vi "QueryFirst.vi"(6 "commandTimeout in":i32=-1, 7 "CommandType":i32(ring)=-1 items=["Text"=1, "StoredProcedure"=4, "TableDirect"=512], 8 "error in (no error)":errorcluster, 9 "DynamicParameters in":refnum<class "DynamicParameters.lvclass">, 10 "sql":string, 11 "ADOMapper in":refnum<class "ADOMapper.lvclass">) -> (0 "error out":errorcluster, 2 "Value":variant, 3 "ADOMapper out":refnum<class "ADOMapper.lvclass">)   [LabVIEW 2020, in "ORM_ADONet.lvlib" / "ADOMapper.lvclass"]
uses:
  ADOMapper.lvclass
  C:/Program Files/National Instruments/LabVIEW 2020/vi.lib/Viviota/shared/ORM.lvlibp/ORM/SqlMapper/SqlMapper.lvclass
  <vilib>/Viviota/shared/ORM.lvlibp/ORM/DynamicParameters/DynamicParameters.lvclass
  <vilib>/Viviota/shared/ORM_DBC_dotNet.lvlibp/dbcDotNet/ORM_DBC_dotNet.lvclass
  System.Data
  <vilib>/Viviota/shared/ORM.lvlibp/ORM/SqlMapper/Read DbConnection.vi
  <vilib>/Viviota/shared/ORM_DBC_dotNet.lvlibp/dbcDotNet/Read transaction.vi
  <vilib>/Viviota/shared/ORM.lvlibp/ORM/DbConnection/DbConnection.lvclass
  ADORow/ADORow.lvclass
  <userlib>/_OpenG.lib/error/error.llb/openg_error.lvlib
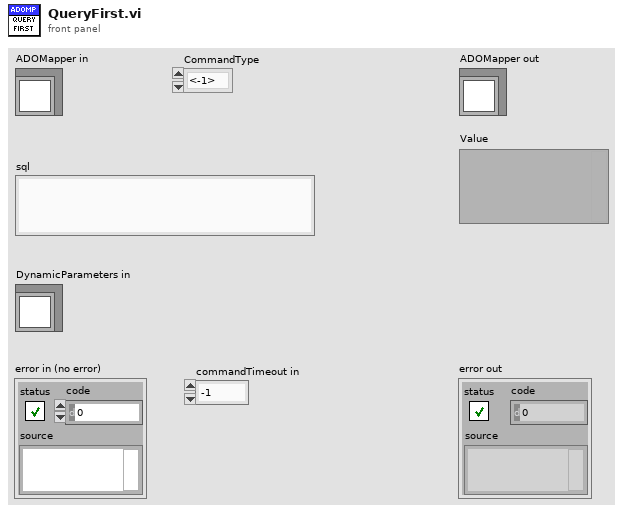
[diagram p1: front panel]
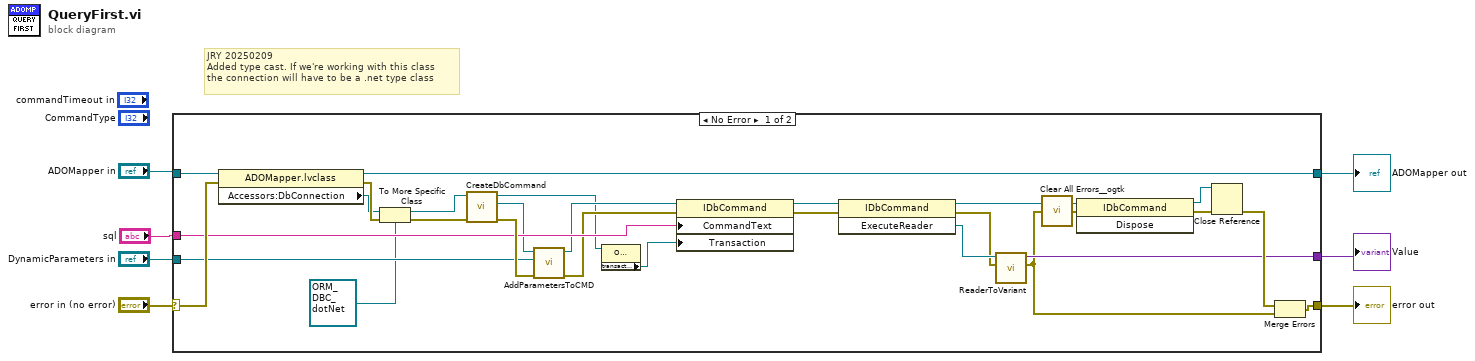
[diagram p0: block diagram]
diagram:
  # "JRY 20250209\nAdded type cast. If we're working with this class\nthe connection will have to be a .net type class"
  n1 = case shown="No Error" "error in (no error)" {
    selector: "error in (no error)" -> [w33 w37]
    tunnel: "ADOMapper in" -> [w35 w36]
    tunnel: [w34 w36] -> w3
    tunnel: "sql" -> [w30 _]
    tunnel: [w15 w37] -> w2
    tunnel: "DynamicParameters in" -> [w21 _]
    tunnel: [w18 _] -> w1
    frame No Error {
      n2 = property class="ADOMapper.lvclass"(reference=w35, error in=w33) -> (reference out=w34:refnum<class "ADOMapper.lvclass">, error out=w32:errorcluster, "Accessors:DbConnection"=w10:refnum<class "DbConnection.lvclass">)
      n3 = To More Specific Class(target class=refnum<class "ORM_DBC_dotNet.lvclass"> refnum ("ORM_DBC_dotNet.lvlibp:ORM_DBC_dotNet.lvclass"), reference=w10, error in=w32) -> (specific class reference=w9:refnum<class "ORM_DBC_dotNet.lvclass">, error out=w11:errorcluster)
      n4 = call <vilib>:"CreateDbCommand.vi"("error in (no error)"=w11, "DbConnection in"=w9) -> ("error out"=w31:errorcluster, "CreateCommand"=w22:refnum<k24>, "DbConnection out"=w17:refnum<class "ORM_DBC_dotNet.lvclass">)  [unwired: 7 in]
      n5 = call "AddParametersToCMD.vi"("error in (no error)"=w31, "DynamicParameters in"=w21, "CreateCommand"=w22) -> ("error out"=w28:errorcluster, "CreateCommand Out"=w20:refnum<k24>)  [unwired: 7 in]
      n6 = property class="ORM_DBC_dotNet.lvclass"(reference=w17) -> ("transaction"=w12:refnum<k24>)  [unwired: 1 in, 2 out]
      n7 = property class="IDbCommand"(reference=w20, error in=w28, "CommandText"=w30, "Transaction"=w12) -> (reference out=w29:refnum<k24>, error out=w26:errorcluster)
      n8 = invoke class="IDbCommand" method="ExecuteReader"(reference=w29, error in=w26) -> (reference out=w25:refnum<k24>, error out=w19:errorcluster, "ExecuteReader"=w27:refnum<k24>)  [unwired: 1 in]
      n9 = call "ReaderToVariant.vi"("Error In"=w19, "Reader"=w27) -> ("Error Out"=w14:errorcluster, "Variant"=w18:variant)  [unwired: 7 in, 1 out]
      n10 = call <userlib>:"Clear All Errors__ogtk.vi"("Error In"=w14) -> ("Error Out"=w16:errorcluster)  [unwired: 3 in]
      n11 = invoke class="IDbCommand" method="Dispose"(reference=w25, error in=w16) -> (reference out=w23:refnum<k24>, error out=w13:errorcluster)  [unwired: 1 in, 1 out]
      n12 = Close Reference(reference=w23, error in (no error)=w13) -> (error out=w24:errorcluster)
      n13 = Merge Errors(w24, w14) -> (w15:errorcluster)
    }
    frame Error {
    }
  }
  "error out" <- w2
  "ADOMapper out" <- w3
  "Value" <- w1
